vi "DataAquisition.vi"() -> ()   [LabVIEW 2020]
uses:
  Readings.vi
  <vilib>/DAQmx/read.llb/DAQmx Read (Analog 1D DBL NChan 1Samp).vi
panel:
  out "Task error out":errorcluster
  in  "stop":bool
  in  "DAQmx Task Name":refnum<k21>
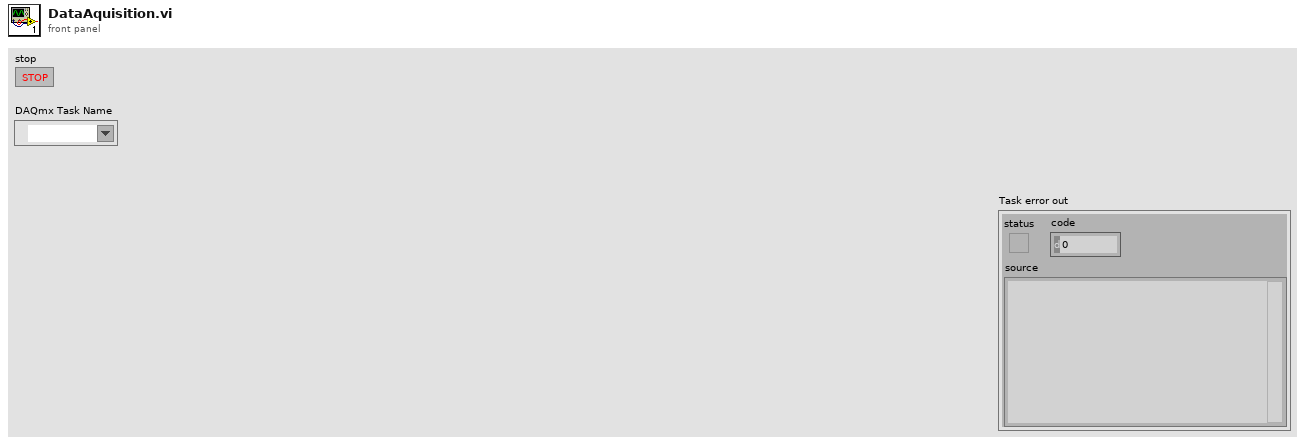
[diagram p1: front panel]
types:
  T1 = cluster{"data[0]":dbl, "data[1]":dbl, "data[2]":dbl, "data[3]":dbl, "data[4]":dbl, "data[5]":dbl, "data[6]":dbl, "data[7]":dbl, "data[8]":dbl}
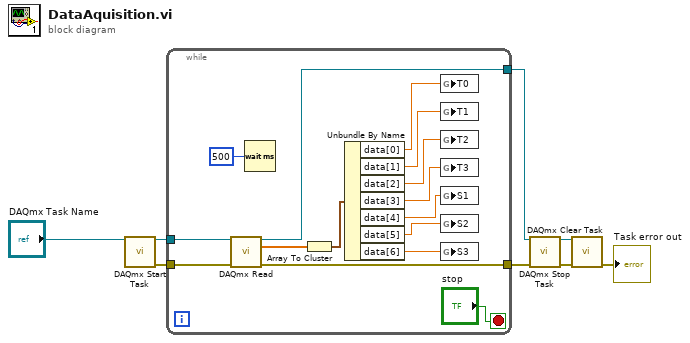
[diagram p0: block diagram]
diagram:
  n1 = call <vilib>:"DAQmx Start Task.vi"("task/channels in"="DAQmx Task Name") -> ("task out"=w7:refnum<k21>, "error out"=w6:errorcluster)  [unwired: 13 in]
  n2 = while {
    tunnel: w7 -> [w22]
    tunnel: w6 -> [w21]
    tunnel: [w19] -> w2
    tunnel: [w18] -> w1
    stop <- "stop" stop-if-true
    n3 = call-poly <vilib>:"DAQmx Read.vi"("task/channels in"=w22, "error in"=w21) -> ("task out"=w18:refnum<k21>, "data"=w20:dbl[], "error out"=w19:errorcluster)  [unwired: 11 in]
    n4 = Wait (ms)(milliseconds to wait=u32 500) -> ()  [unwired: 1 out]
    n5 = Array To Cluster(array=w20) -> (cluster=w17:T1)
    n6 = Unbundle By Name(w17) -> ("data[0]"=w15:dbl, "data[1]"=w14:dbl, "data[2]"=w13:dbl, "data[3]"=w12:dbl, "data[4]"=w11:dbl, "data[5]"=w10:dbl, "data[6]"=w9:dbl)
    n7 = global write "Readings.vi" "T0"(w15) -> ()
    n8 = global write "Readings.vi" "T1"(w14) -> ()
    n9 = global write "Readings.vi" "T2"(w13) -> ()
    n10 = global write "Readings.vi" "T3"(w12) -> ()
    n11 = global write "Readings.vi" "S1"(w11) -> ()
    n12 = global write "Readings.vi" "S2"(w10) -> ()
    n13 = global write "Readings.vi" "S3"(w9) -> ()
  }
  n14 = call <vilib>:"DAQmx Stop Task.vi"("task/channels in"=w1, "error in"=w2) -> ("task out"=w5:refnum<k21>, "error out"=w4:errorcluster)  [unwired: 12 in]
  n15 = call <vilib>:"DAQmx Clear Task.vi"("task in"=w5, "error in"=w4) -> ("error out"=→"Task error out":errorcluster)  [unwired: 13 in]
